vi "Export_mappingFileName.vi"(0 "ITC503 Current Values":T3 {"ITC503 Gradient" format="%.2f"; "ITC503 Setpoint" min=-273.0 max=300000.0 step=0.0001 format="%.1f"; "ITC503 I" format="%_1f"; "ITC503 P" format="%_1f"; "ITC503 Temperature" min=0.0 max=1645.0 step=1e-05 format="%.2f"; "ITC503 Heater" min=0.0 max=100.0 step=0.01 scale=0.0..100.0}, 1 "iHR Current Values":T4={"iHR 550 Front Entrance"=0.0, "iHR550 Side Exit"=0.0, "iHR550 Wavelength"=897.9988, "iHR550 Exit Mirror"=2, "iHR550 Grating"="1", "Grating Index"=1} {"iHR550 Exit Mirror" items=["EntranceMirror", "ExitMirror", "Front", "Side"]}, 2 "Spectra Settings":T2={"Integration Time"=10.0, "Repetitions"=10, "Mapping Spectra"=TRUE} caption="Mapping Spectra Settings" {"Repetitions" min=1 max=100 step=1; "Integration Time" min=0.5 max=6000.0 step=1.0 format="%.1f"}, 3 "Mapping Parameters":T1={"X Start Position"=0.0, "X Stop Position"=10.0, "Y Start Position"=0.0, "Y Stop Position"=10.0, "Step Size"=1.0} {"Step Size" min=0.1 max=30.0 step=0.1 format="%.1f"; "Y Stop Position" min=0.0 max=30.0 step=0.1 format="%.1f"; "Y Start Position" min=0.0 max=30.0 step=0.1 format="%.1f"; "X Stop Position" min=0.0 max=30.0 step=0.1 format="%.1f"; "X Start Position" min=0.0 max=30.0 step=0.1 format="%.1f"}, 4 "CCD3500 Temperature":dbl caption="Temp. (°C)" min=10.0 max=160.0 step=0.1 format="%.1f") -> (5 "Filename":string)   [LabVIEW 2010]
uses:
  iHR550/TypeDefs/iHR Current Values.ctl
  ITC503/TypeDefs/ITC503 Current Values.ctl
  Mapping/TypeDefs/Mapping Spectra Params.ctl
  Mapping/TypeDefs/Mapping Drive Params.ctl
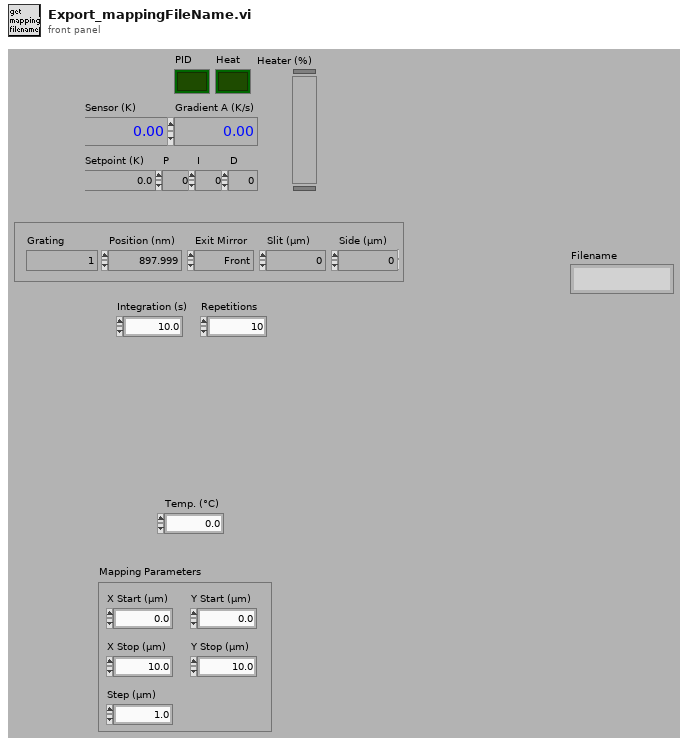
[diagram p1: front panel]
types:
  T1 = typedef "Mapping Drive Params.ctl" = cluster{"X Start Position":dbl, "X Stop Position":dbl, "Y Start Position":dbl, "Y Stop Position":dbl, "Step Size":dbl}
  T2 = typedef "Mapping Spectra Params.ctl" = cluster{"Integration Time":dbl, "Repetitions":u16, "Mapping Spectra":bool}
  T3 = typedef "ITC503 Current Values.ctl" = cluster{"ITC503 Heater":dbl, "ITC503 Temperature":dbl, "ITC503 P":dbl, "ITC503 I":dbl, "ITC503 D":dbl, "ITC503 Setpoint":dbl, "ITC503 Gradient":dbl, "ITC503 Heater Auto":bool, "ITC503 PID Auto":bool}
  T4 = typedef "iHR Current Values.ctl" = cluster{"iHR 550 Front Entrance":dbl, "iHR550 Side Exit":dbl, "iHR550 Wavelength":dbl, "iHR550 Exit Mirror":i32, "iHR550 Grating":string, "Grating Index":i32}
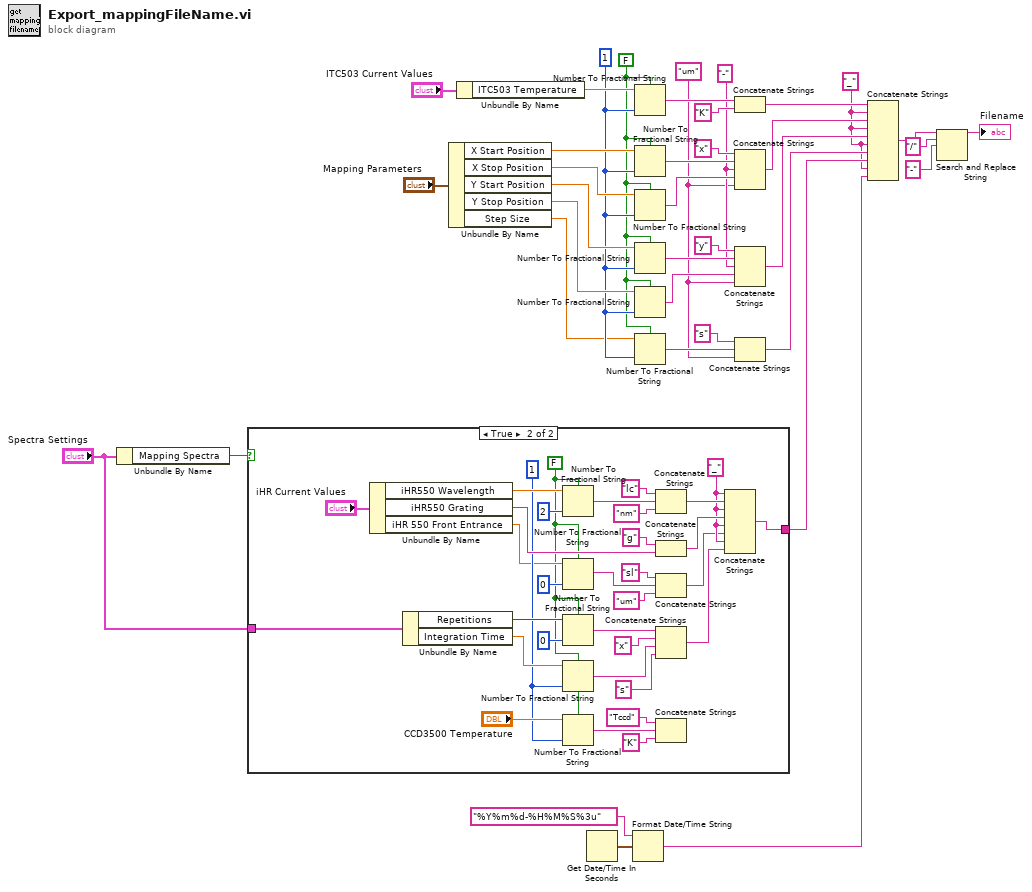
[diagram p0: block diagram]
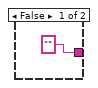
[diagram p2: hidden frame]
diagram:
  w17 = "-" ("string")
  w1 = "_" ("String")
  w11 = "um" ("String")
  w14 = FALSE ("Systemdezimalzeichen verwenden (T)")
  w15 = i16 1 ("Genauigkeit (6)")
  n1 = Unbundle By Name("Spectra Settings") -> ("Mapping Spectra"=w23:bool)
  n2 = case shown="True" w23 {
    tunnel: "Spectra Settings" -> [_ w52]
    tunnel: ["" w48] -> w6
    frame False {
    }
    frame True {
      w47 = "_" ("String")
      w42 = FALSE ("use system decimal point (T)")
      w51 = i16 1 ("precision (6)")
      n3 = Unbundle By Name("iHR Current Values") -> ("iHR550 Wavelength"=w69:dbl, "iHR550 Grating"=w54:string, "iHR 550 Front Entrance"=w44:dbl)
      n4 = Unbundle By Name(w52) -> ("Repetitions"=w70:u16, "Integration Time"=w61:dbl)
      n5 = Number To Fractional String(use system decimal point (T)=w42, number=w69, precision (6)=i16 2 ("Genauigkeit (6)")) -> (F-format string=w57:string)  [unwired: 1 in]
      n6 = Number To Fractional String(use system decimal point (T)=w42, number=w44, precision (6)=i16 0 ("Genauigkeit (6)")) -> (F-format string=w41:string)  [unwired: 1 in]
      n7 = Number To Fractional String(use system decimal point (T)=w42, number=w70, precision (6)=i16 0 ("Genauigkeit (6)")) -> (F-format string=w64:string)  [unwired: 1 in]
      n8 = Number To Fractional String(use system decimal point (T)=w42, number=w61, precision (6)=w51) -> (F-format string=w63:string)  [unwired: 1 in]
      n9 = Number To Fractional String(use system decimal point (T)=w42, number="CCD3500 Temperature", precision (6)=w51) -> (F-format string=w60:string)  [unwired: 1 in]
      n10 = Concatenate Strings("lc" ("String"), w57, "nm" ("String")) -> (w50:string)
      n11 = Concatenate Strings("g" ("String"), w54) -> (w49:string)
      n12 = Concatenate Strings("sl" ("String"), w41, "um" ("String")) -> (w39:string)
      n13 = Concatenate Strings(w64, "x" ("String"), w63, "s" ("String")) -> (w40:string)
      n14 = Concatenate Strings("Tccd" ("String"), w60, "K" ("String")) -> ()  [unwired: 1 out]
      n15 = Concatenate Strings(w47, w50, w47, w49, w47, w39, w47, w40) -> (w48:string)
    }
  }
  n16 = Unbundle By Name("Mapping Parameters") -> ("X Start Position"=w35:dbl, "X Stop Position"=w22:dbl, "Y Start Position"=w19:dbl, "Y Stop Position"=w20:dbl, "Step Size"=w13:dbl)
  n17 = Unbundle By Name("ITC503 Current Values") -> ("ITC503 Temperature"=w36:dbl)
  n18 = Get Date/Time In Seconds() -> (seconds since 1Jan1904=w4:timestamp)
  n19 = Format Date/Time String(time format string (%c)="%Y%m%d-%H%M%S%3u", seconds (now)=w4) -> (date/time string=w2:string)  [unwired: 1 in]
  n20 = Number To Fractional String(use system decimal point (T)=w14, number=w36, precision (6)=w15) -> (F-format string=w34:string)  [unwired: 1 in]
  n21 = Number To Fractional String(use system decimal point (T)=w14, number=w35, precision (6)=w15) -> (F-format string=w32:string)  [unwired: 1 in]
  n22 = Number To Fractional String(use system decimal point (T)=w14, number=w22, precision (6)=w15) -> (F-format string=w21:string)  [unwired: 1 in]
  n23 = Number To Fractional String(use system decimal point (T)=w14, number=w19, precision (6)=w15) -> (F-format string=w31:string)  [unwired: 1 in]
  n24 = Number To Fractional String(use system decimal point (T)=w14, number=w20, precision (6)=w15) -> (F-format string=w18:string)  [unwired: 1 in]
  n25 = Number To Fractional String(use system decimal point (T)=w14, number=w13, precision (6)=w15) -> (F-format string=w12:string)  [unwired: 1 in]
  n26 = Concatenate Strings(w34, "K" ("String")) -> (w10:string)
  n27 = Concatenate Strings("x" ("String"), w32, w17, w21, w11) -> (w9:string)
  n28 = Concatenate Strings("y" ("String"), w31, w17, w18, w11) -> (w8:string)
  n29 = Concatenate Strings("s" ("String"), w12, w11) -> (w7:string)
  n30 = Concatenate Strings(w10, w1, w9, w1, w8, w1, w7, w6, w1, w2) -> (w28:string)
  n31 = Search and Replace String(input string=w28, search string="/" ("Such-String"), replace string="-" ("replace string (\"\")")) -> (result string=→"Filename":string)  [unwired: 5 in, 3 out]
